vi "Try Lookup Telemetry API.vi"(8 "error in (no error)":errorcluster, 11 "Task in":refnum<class "Task.lvclass">) -> (0 "error out":errorcluster, 3 "Task out":refnum<class "Task.lvclass">)   [LabVIEW 2020, in "Volatus.lvlib" / "Task.lvclass"]
uses:
  Task.lvclass
  TelemetryAPI/TelemetryAPI.lvclass
  C:/dev/lv20CE/relink/lv-volatus/Volatus/API/API.lvclass
  Task.lvclass/Task.ctl
  VolatusAPI/VolatusAPI.lvclass/VolatusAPI.ctl
  Identity/Key.vi
  <vilib>/Utility/error.llb/Error Cluster From Error Code.vi
  API/API.lvclass
  Identity/Identity.lvclass
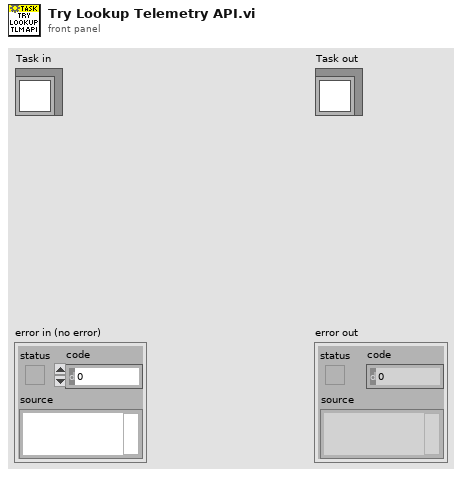
[diagram p1: front panel]
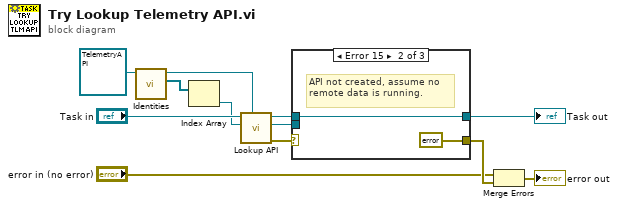
[diagram p0: block diagram]
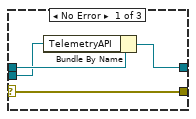
[diagram p2: hidden frame]
diagram:
  n1 = call-dynamic "Identities.vi"("TelemetryAPI in"=refnum<class "TelemetryAPI.lvclass"> refnum ("Volatus:TelemetryAPI")) -> ("Identities"=w9:refnum<class "Identity.lvclass">[], "TelemetryAPI out"=w10:refnum<class "TelemetryAPI.lvclass">)  [unwired: 8 in, 1 out]
  n2 = Index Array(array=w9) -> (element=w8:refnum<class "Identity.lvclass">)  [unwired: 1 in]
  n3 = call "Lookup API.vi"("API Type"=w10, "Identity"=w8, "Task in"="Task in") -> ("error out"=w7:errorcluster, "API"=w6:refnum<class "TelemetryAPI.lvclass">, "Task out"=w5:refnum<class "Task.lvclass">)  [unwired: 6 in]
  n4 = case shown="Error 15" w7 {
    selector: w7 -> [w13 _ w20]
    tunnel: w6 -> [w15 _ _]
    tunnel: w5 -> [w16 w18 w19]
    tunnel: [w14 w18 w19] -> w4
    tunnel: [w13 errorcluster {"status"=FALSE, "code"=0, "source"=""} ("error IO") w20] -> w3
    frame No Error {
      n5 = Bundle By Name(cluster=w16, "TelemetryAPI"=w15) -> (w14:refnum<class "Task.lvclass">)
    }
    frame Error {
      # "API not created, assume no remote data is running."
    }
    frame Default {
      # "Unknown error"
    }
  }
  "Task out" <- w4
  n6 = Merge Errors("error in (no error)", w3) -> (→"error out":errorcluster)
